vi "Check-displacement.vi"(8 "error in (no error)":errorcluster, 10 "Displacement in":dbl caption="Displacement [unit]", 11 "Motor-Serial in":refnum<class "Motor-Analog.lvclass">) -> (0 "error out":errorcluster, 1 "In range?":bool, 2 "Displacement out":dbl caption="Displacement out [unit]", 3 "Motor-Serial out":refnum<class "Motor-Analog.lvclass">)   [LabVIEW 2013, in "PowderDeposition.lvlib" / "Motor-Analog.lvclass"]
uses:
  Motor-Analog.lvclass
  Motor-Analog.lvclass/Motor-Analog.ctl
  Read Maximum value.vi
  Read Minimum value.vi
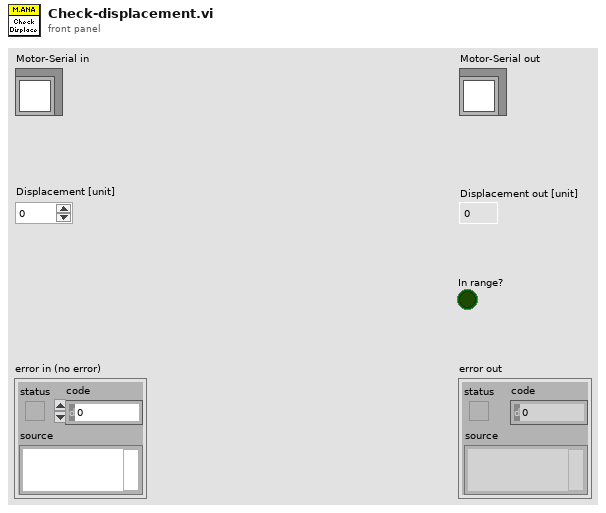
[diagram p1: front panel]
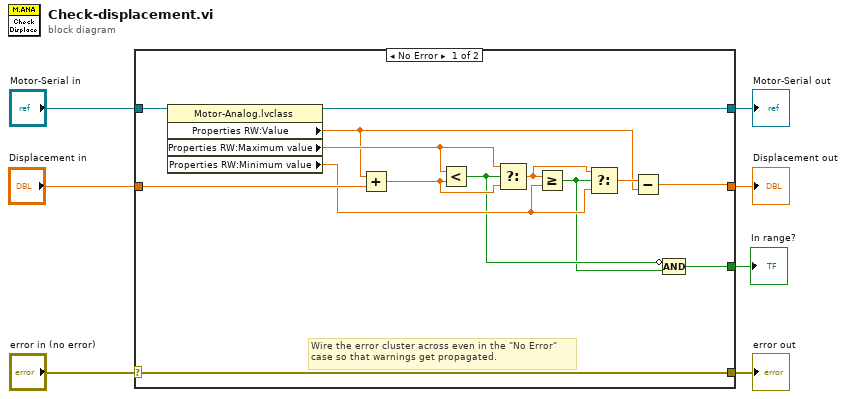
[diagram p0: block diagram]
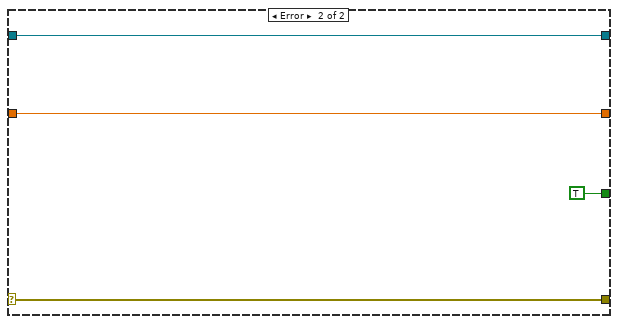
[diagram p2: hidden frame]
diagram:
  n1 = case shown="No Error" "error in (no error)" {
    selector: "error in (no error)" -> [w20 w25]
    tunnel: [w20 w25] -> w6
    tunnel: [w19 w24] -> w4
    tunnel: "Motor-Serial in" -> [w21 w24]
    tunnel: "Displacement in" -> [w18 w23]
    tunnel: [w10 w23] -> w2
    tunnel: [w8 TRUE] -> w1
    frame No Error {
      # "Wire the error cluster across even in the \"No Error\"\ncase so that warnings get propagated."
      n2 = property class="Motor-Analog.lvclass"(reference=w21) -> (reference out=w19:refnum<class "Motor-Analog.lvclass">, "Properties RW:Value"=w11:dbl, "Properties RW:Maximum value"=w17:dbl, "Properties RW:Minimum value"=w15:dbl)  [unwired: 1 in, 1 out]
      n3 = Add(x=w11, y=w18) -> (x+y=w16:dbl)
      n4 = Less?(x=w17, y=w16) -> (x < y?=w13:bool)
      n5 = Select(t=w17, s=w13, f=w16) -> (s? t:f=w14:dbl)
      n6 = Greater Or Equal?(x=w14, y=w15) -> (x >= y?=w9:bool)
      n7 = Select(t=w14, s=w9, f=w15) -> (s? t:f=w12:dbl)
      n8 = Subtract(x=w12, y=w11) -> (x-y=w10:dbl)
      n9 = Compound Arithmetic op=AND(invert w13, w9) -> (w8:bool)
    }
    frame Error {
    }
  }
  "error out" <- w6
  "Motor-Serial out" <- w4
  "Displacement out" <- w2
  "In range?" <- w1
